vi "Head Tail Detection Angle Based (HOST).vi"() -> ()   [LabVIEW 2015]
uses:
  <vilib>/Analysis/baseanly.llb/Mean (DBL).vi
  <vilib>/vision/NI_Vision_Development_Module.lvlib
  <vilib>/Analysis/NI_AALBase.lvlib
panel:
  in  "Frame #":i32=40
  out "Frame #":i32
  in  "Loop Interval":u32=1000
  in  "Stop Button":bool
  out "Array (HOST)":i32[](array[numeric])
  out "Dip (HOST)":i16[](graph)
  out "Angle (HOST)":dbl[](graph)
  out "# of Contour Points":i32
  out "Contour":cluster{u16[], u16[]}(graph)
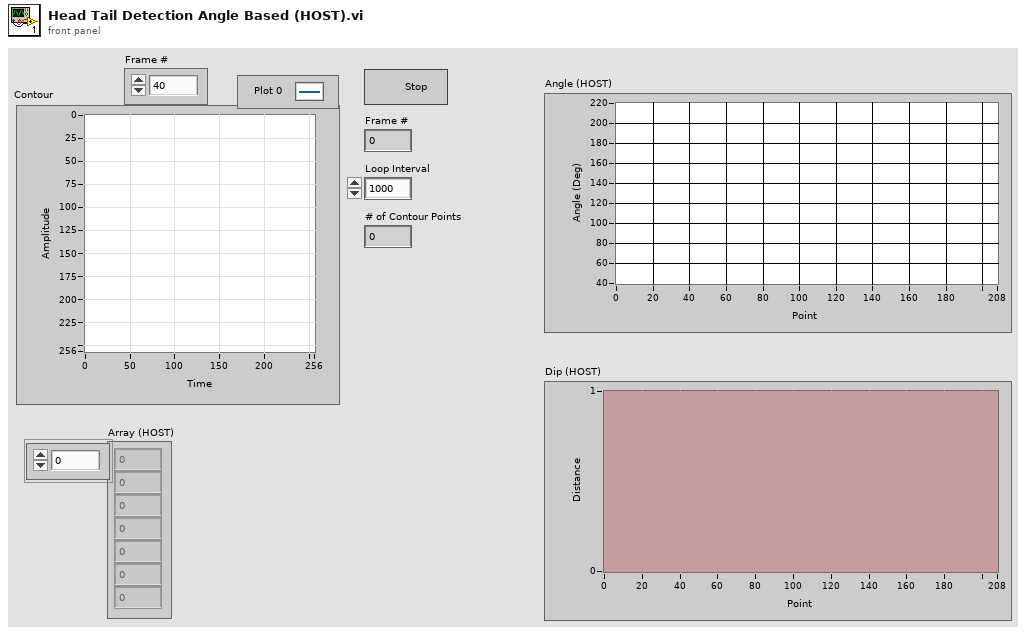
[diagram p1: front panel]
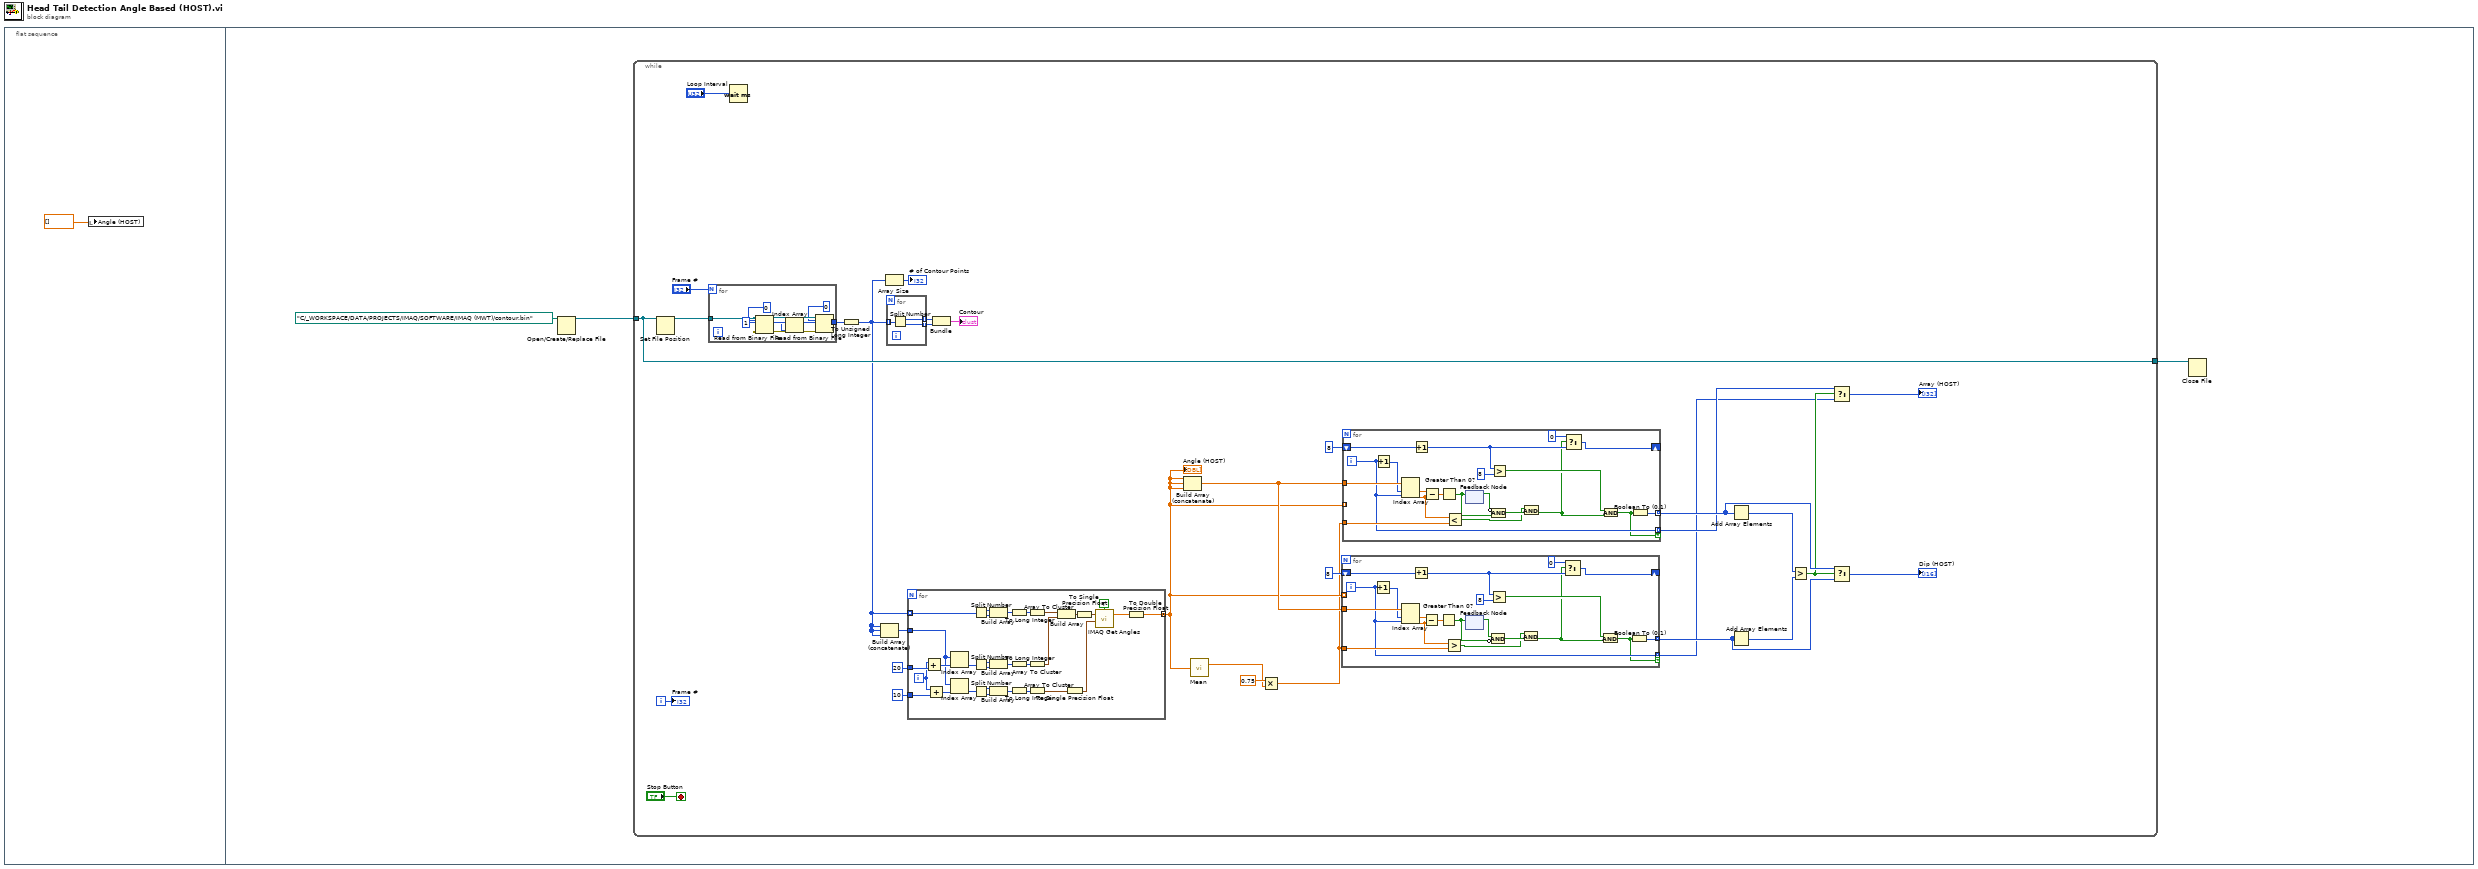
[diagram p0: block diagram]
diagram:
  n1 = flat-sequence {
    frame #0 {
      n2 = local write "Angle (HOST)"(dbl[] []) -> ()
    }
    frame #1 {
      n3 = Open/Create/Replace File(file path (use dialog)=path "C:/_WORKSPACE/DATA/PROJECTS/IMAQ/SOFTWARE/IMAQ (MWT)/contour.bin") -> (refnum out=w4:refnum<file>)  [unwired: 5 in, 2 out]
      n4 = while {
        tunnel: w4 -> [w34]
        tunnel: [w34] -> w3
        i -> [w29]
        stop <- "Stop Button" stop-if-true
        n5 = Set File Position(refnum=w34) -> (refnum out=w28:refnum<file>)  [unwired: 3 in, 1 out]
        n6 = for {
          N: "Frame #" -> [_]
          tunnel: w28 -> [w44]
          tunnel: [w36] -> w11
          n7 = Read from Binary File(5:0 ("count (1)"), 10:1 ("count (1)"), 11:w44) -> (0:w42:errorcluster, 2:w39:i32[], 3:w41:refnum<file>)  [unwired: 3 in, 1 out]
          n8 = Index Array(array=w39) -> (element=w38:i32)  [unwired: 1 in]
          n9 = Read from Binary File(5:u32 0 ("count (1)"), 8:w42, 10:w38, 11:w41) -> (2:w36:u32[])  [unwired: 2 in, 3 out]
        }
        n10 = Wait (ms)(milliseconds to wait="Loop Interval") -> ()  [unwired: 1 out]
        n11 = To Unsigned Long Integer(number=w11) -> (unsigned 32bit integer=w15:u32[])
        n12 = Build Array (concatenate)(w15, w15, w15) -> (w14:u32[])
        n13 = Array Size(array=w15) -> (size(s)=→"# of Contour Points":i32)
        n14 = for {
          tunnel: w15 -> [w87] mode=indexing
          tunnel: [w86] -> w31 mode=indexing
          tunnel: [w85] -> w32 mode=indexing
          n15 = Split Number(x=w87) -> (hi(x)=w86:u16, lo(x)=w85:u16)
        }
        n16 = for {
          tunnel: w15 -> [w115] mode=indexing
          tunnel: w14 -> [w98]
          tunnel: 20 -> [w113]
          tunnel: 10 -> [w112]
          tunnel: [w94] -> w8 mode=concatenating
          i -> [w111]
          n17 = Add(x=w111, y=w113) -> (x+y=w106:i32)
          n18 = Add(x=w111, y=w112) -> (x+y=w99:i32)
          n19 = Index Array(array=w98, index=w106) -> (element=w110:u32)
          n20 = Index Array(array=w98, index=w99) -> (element=w100:u32)
          n21 = Split Number(x=w115) -> (hi(x)=w117:u16, lo(x)=w116:u16)
          n22 = Split Number(x=w110) -> (hi(x)=w108:u16, lo(x)=w107:u16)
          n23 = Split Number(x=w100) -> (hi(x)=w102:u16, lo(x)=w103:u16)
          n24 = Build Array(w117, w116) -> (w114:u16[])
          n25 = Build Array(w108, w107) -> (w109:u16[])
          n26 = Build Array(w102, w103) -> (w101:u16[])
          n27 = To Long Integer(number=w114) -> (32bit integer=w89:i32[])
          n28 = To Long Integer(number=w109) -> (32bit integer=w88:i32[])
          n29 = To Long Integer(number=w101) -> (32bit integer=w90:i32[])
          n30 = Array To Cluster(array=w89) -> (cluster=w91:cluster{"[0]":i32, "[1]":i32})
          n31 = Array To Cluster(array=w88) -> (cluster=w92:cluster{"[0]":i32, "[1]":i32})
          n32 = Array To Cluster(array=w90) -> (cluster=w93:cluster{"[0]":i32, "[1]":i32})
          n33 = Build Array(w91, w92) -> (w105:cluster{"[0]":i32, "[1]":i32}[])
          n34 = To Single Precision Float(number=w93) -> (single precision float=w97:cluster{"[0]":sgl, "[1]":sgl})
          n35 = To Single Precision Float(number=w105) -> (single precision float=w104:cluster{"[0]":sgl, "[1]":sgl}[])
          n36 = call "IMAQ Get Angles"("Vertex"=w97, "Points"=w104, "Use Vertex (No)"=TRUE) -> ("Angles (deg)"=w96:sgl[])  [unwired: 2 in, 2 out]
          n37 = To Double Precision Float(number=w96) -> (double precision float=w94:dbl[])
        }
        "Angle (HOST)" <- w8
        n38 = Bundle(w31, w32) -> (→"Contour":cluster{u16[], u16[]})  [unwired: 1 in]
        n39 = Build Array (concatenate)(w8, w8, w8) -> (w25:dbl[])
        n40 = call-poly <vilib>:"Mean.vi"("X"=w8) -> ("mean"=w6:dbl)  [unwired: 1 out]
        n41 = Multiply(x=0.75, y=w6) -> (x*y=w5:dbl)
        n42 = for {
          tunnel: w25 -> [w64]
          tunnel: [w59] -> w22 mode=indexing
          tunnel: w5 -> [w58]
          shift-right: [w56] -> _
          shift-left: 8 ("x") -> [w57]
          tunnel: w8 -> [_] mode=indexing
          tunnel: [w48] -> w17 mode=indexing if=w47
          i -> [w48]
          n43 = Increment(x=w48) -> (x+1=w50:i32)
          n44 = Index Array(array=w64, index #1=w50, index #2=w48) -> (element #1=w63:dbl, element #2=w49:dbl)
          n45 = Increment(x=w57) -> (x+1=w53:i32)
          n46 = Subtract(x=w63, y=w49) -> (x-y=w62:dbl)
          n47 = Greater Than 0?(x=w62) -> (x > 0?=w60:bool)
          n48 = Greater?(x=w49, y=w58) -> (0:w45:bool)
          n49 = feedback-in #1(w60) -> ()
          n50 = feedback #1() -> (w61:bool)  [unwired: 1 in]
          n51 = Greater?(x=w53, y=8) -> (0:w51:bool)
          n52 = Compound Arithmetic op=AND(w61, invert w60) -> (w54:bool)
          n53 = And(x=w45, y=w54) -> (x .and. y?=w46:bool)
          n54 = Select(t=0, s=w46, f=w53) -> (s? t:f=w56:i32)
          n55 = And(x=w51, y=w46) -> (x .and. y?=w47:bool)
          n56 = Boolean To (0,1)(Boolean=w47) -> (0, 1=w59:i16)
        }
        n57 = for {
          tunnel: w25 -> [w84]
          tunnel: [w79] -> w21 mode=indexing
          tunnel: w8 -> [_] mode=indexing
          tunnel: w5 -> [w78]
          shift-right: [w76] -> _
          shift-left: 8 ("x") -> [w77]
          tunnel: [w68] -> w18 mode=indexing if=w67
          i -> [w68]
          n58 = Increment(x=w68) -> (x+1=w70:i32)
          n59 = Index Array(array=w84, index #1=w70, index #2=w68) -> (element #1=w83:dbl, element #2=w69:dbl)
          n60 = Increment(x=w77) -> (x+1=w73:i32)
          n61 = Subtract(x=w83, y=w69) -> (x-y=w82:dbl)
          n62 = Greater Than 0?(x=w82) -> (x > 0?=w80:bool)
          n63 = Less?(x=w69, y=w78) -> (x < y?=w65:bool)
          n64 = feedback-in #2(w80) -> ()
          n65 = feedback #2() -> (w81:bool)  [unwired: 1 in]
          n66 = Greater?(x=w73, y=8) -> (0:w71:bool)
          n67 = Compound Arithmetic op=AND(invert w81, w80) -> (w74:bool)
          n68 = And(x=w65, y=w74) -> (x .and. y?=w66:bool)
          n69 = Select(t=0, s=w66, f=w73) -> (s? t:f=w76:i32)
          n70 = And(x=w71, y=w66) -> (x .and. y?=w67:bool)
          n71 = Boolean To (0,1)(Boolean=w67) -> (0, 1=w79:i16)
        }
        n72 = Add Array Elements(numeric array=w21) -> (sum=w24:i16)
        n73 = Add Array Elements(numeric array=w22) -> (sum=w23:i16)
        n74 = Greater?(x=w24, y=w23) -> (0:w19:bool)
        n75 = Select(t=w18, s=w19, f=w17) -> (s? t:f=→"Array (HOST)":i32[])
        n76 = Select(t=w21, s=w19, f=w22) -> (s? t:f=→"Dip (HOST)":i16[])
        "Frame #" <- w29
      }
      n77 = Close File(refnum=w3) -> ()  [unwired: 1 in, 2 out]
    }
  }
